vi "HGF_DSCmonitor_register.vi"(0 "HGF_DSCMonitor in":refnum<class "HGF_DSCMonitor.lvclass">, 2 "SV":refnum<k21>, 3 "HGF_NetworkVisitor":refnum<class "HGF_NetworkVisitor.lvclass">, 4 "HGF_TriggeredEvent":refnum<class "HGF_TriggeredEvent.lvclass">, 5 "error in (no error)":errorcluster, 7 "request changes (all changes)":u16(ring) items=["all changes", "value changes only"]) -> (14 "HGF_DSCMonitor out":refnum<class "HGF_DSCMonitor.lvclass">, 19 "error out":errorcluster)   [LabVIEW 2012, in "HGF_DSC.lvlib" / "HGF_DSCMonitor.lvclass"]
uses:
  HGF_DSCMonitor.lvclass
  HGF_BaseClasses/HGF_NetworkVisitor/HGF_NetworkVisitor.lvclass
  HGF_BaseClasses/HGF_TriggeredEvent/HGF_TriggeredEvent.lvclass
  HGF_DSCMonitor.lvclass/HGF_DSCMonitor.ctl
  <vilib>/lvdsc/NI_DSC.lvlib
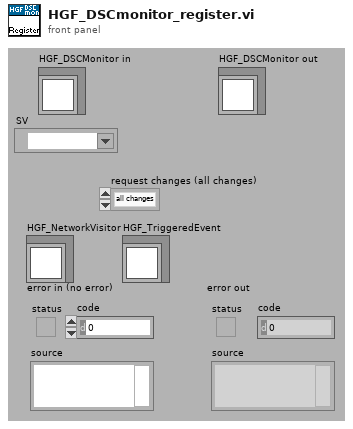
[diagram p1: front panel]
types:
  T1 = cluster{"Shared Variable":refnum<k21>, "registered Visitors":cluster{"HGF_NetworkVisitor":refnum<class "HGF_NetworkVisitor.lvclass">, "HGF_TriggeredEvent":refnum<class "HGF_TriggeredEvent.lvclass">}[]}[]
  T2 = cluster{"Shared Variable":refnum<k21>, "registered Visitors":cluster{"HGF_NetworkVisitor":refnum<class "HGF_NetworkVisitor.lvclass">, "HGF_TriggeredEvent":refnum<class "HGF_TriggeredEvent.lvclass">}[]}
  T3 = cluster{"HGF_NetworkVisitor":refnum<class "HGF_NetworkVisitor.lvclass">, "HGF_TriggeredEvent":refnum<class "HGF_TriggeredEvent.lvclass">}[]
  T4 = cluster{"HGF_NetworkVisitor":refnum<class "HGF_NetworkVisitor.lvclass">, "HGF_TriggeredEvent":refnum<class "HGF_TriggeredEvent.lvclass">}
  T5 = cluster{"SV":refnum<k21>, cluster{"HGF_NetworkVisitor":refnum<class "HGF_NetworkVisitor.lvclass">, "HGF_TriggeredEvent":refnum<class "HGF_TriggeredEvent.lvclass">}[]}
  T6 = cluster{"SV":refnum<k21>, "registered Visitors":cluster{"HGF_NetworkVisitor":refnum<class "HGF_NetworkVisitor.lvclass">, "HGF_TriggeredEvent":refnum<class "HGF_TriggeredEvent.lvclass">}[]}[]
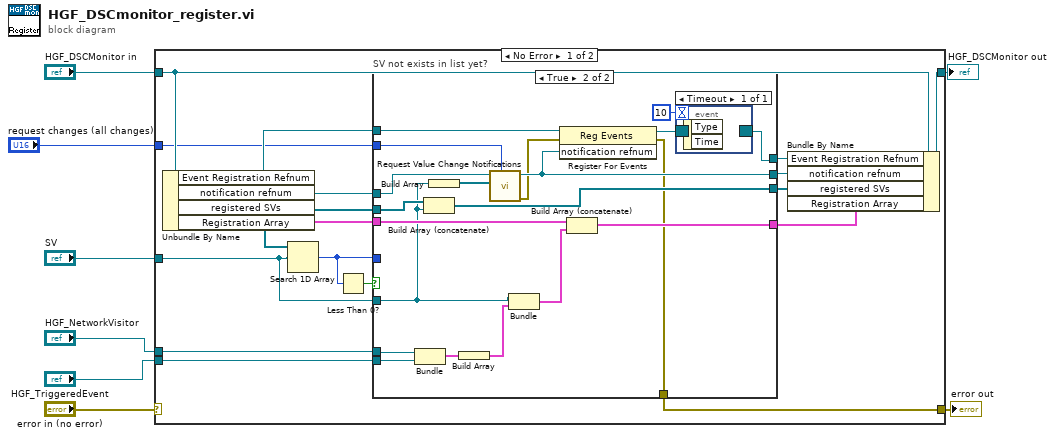
[diagram p0: block diagram]
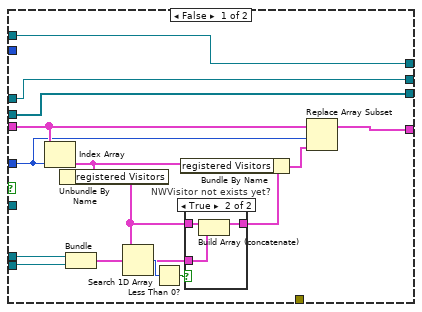
[diagram p2: hidden frame]
diagram:
  n1 = case shown="No Error" "error in (no error)" {
    selector: "error in (no error)" -> [_ w66]
    tunnel: [w9 w66] -> w5
    tunnel: [w21 w65] -> w7
    tunnel: "HGF_DSCMonitor in" -> [w25 w65]
    tunnel: "SV" -> [w11 _]
    tunnel: "HGF_NetworkVisitor" -> [w13 _]
    tunnel: "HGF_TriggeredEvent" -> [w12 _]
    tunnel: "request changes (all changes)" -> [w10 _]
    frame No Error {
      n2 = Unbundle By Name(w25) -> ("Event Registration Refnum"=w16:refnum<event-registration>, "notification refnum"=w22:refnum<user-event>, "registered SVs"=w14:refnum<k21>[], "Registration Array"=w15:T1)
      n3 = Search 1D Array(1D array=w14, element=w11) -> (index of element=w23:i32)  [unwired: 1 out]
      n4 = Less Than 0?(x=w23) -> (x < 0?=w24:bool)
      n5 = case "SV not exists in list yet?" shown="True" w24 {
        tunnel: w13 -> [w39 w61]
        tunnel: w15 -> [w32 w63]
        tunnel: w23 -> [w29 _]
        tunnel: [w31 w58] -> w18
        tunnel: w14 -> [w40 w62]
        tunnel: w11 -> [_ w55]
        tunnel: [w40 w56] -> w19
        tunnel: w22 -> [w28 w57]
        tunnel: [w28 w54] -> w20
        tunnel: [w27 w48] -> w17
        tunnel: w16 -> [w27 w47]
        tunnel: w12 -> [w26 w53]
        tunnel: w10 -> [_ w51]
        tunnel: [_ w45] -> w9
        frame False {
          n6 = Index Array(array=w32, index=w29) -> (element=w34:T2)
          n7 = Unbundle By Name(w34) -> ("registered Visitors"=w35:T3)
          n8 = Bundle("HGF_NetworkVisitor"=w39, "HGF_TriggeredEvent"=w26) -> (w36:T4)  [unwired: 1 out]
          n9 = Search 1D Array(1D array=w35, element=w36) -> (index of element=w38:i32)  [unwired: 1 out]
          n10 = Less Than 0?(x=w38) -> (x < 0?=w37:bool)
          n11 = case "NWVisitor not exists yet?" shown="True" w37 {
            tunnel: w36 -> [_ w43]
            tunnel: w35 -> [w41 w44]
            tunnel: [w41 w42] -> w33
            frame False {
            }
            frame True {
              n12 = Build Array (concatenate)(w44, w43) -> (w42:T3)
            }
          }
          n13 = Bundle By Name(cluster=w34, "registered Visitors"=w33) -> (w30:T2)
          n14 = Replace Array Subset(array=w32, new element=w30, index=w29) -> (w31:T1)
        }
        frame True {
          n15 = Bundle("HGF_NetworkVisitor"=w61, "HGF_TriggeredEvent"=w53) -> (w60:T4)  [unwired: 1 out]
          n16 = Build Array (concatenate)(w62, w55) -> (w56:refnum<k21>[])
          n17 = Build Array(w55) -> (w64:refnum<k21>[])
          n18 = Build Array(w60) -> (w59:T3)
          n19 = call <vilib>:"Request Value Change Notifications.vi"("request changes (all changes)"=w51, "shared variables"=w64, "notification refnum"=w57) -> ("error out"=w46:errorcluster, "shared variable value change notification"=w54:refnum<user-event>)  [unwired: 1 in, 6 out]
          n20 = Bundle("SV"=w55, w59) -> (w52:T5)  [unwired: 1 out]
          n21 = register-events(reference=w47, error in=w46, w54) -> (reference out=w50:refnum<event-registration>, error out=w45:errorcluster)
          n22 = Build Array (concatenate)(w63, w52) -> (w58:T6)
          n23 = event shown="[0] Timeout" {
            selector: w50 -> [_]
            dyn-events: [_] -> w48
            timeout: 10 -> [_]
            event Timeout {
              n24 = event-data() -> ()  [unwired: 3 out]
            }
          }
        }
      }
      n25 = Bundle By Name(cluster=w25, "Event Registration Refnum"=w17, "notification refnum"=w20, "registered SVs"=w19, "Registration Array"=w18) -> (w21:refnum<class "HGF_DSCMonitor.lvclass">)
    }
    frame Error {
    }
  }
  "error out" <- w5
  "HGF_DSCMonitor out" <- w7
